vi "CSM - Read Cluster Elements From Session.vi"(5 "Section Name(\"\" as Default)":string, 8 "error in (no error)":errorcluster, 9 "Cluster":variant) -> (2 "error out":errorcluster, 3 "Cluster out":variant)   [LabVIEW 2017, in "INI-Static-Variable-Support.lvlib"]
uses:
  _Support/_fgv-oper.ctl
  99de0c97-112a-4c86-9094-c187659127e1.vi
  <userlib>/_NEVSTOP/Communicable State Machine(CSM)/addons/API-String-Arugments-Support/_Support/Data To API String Arguments.vi
  INI-Static-Variable-Support.lvlib
  <userlib>/_NEVSTOP/Communicable State Machine(CSM)/addons/API-String-Arugments-Support/API String Arguments Support.lvlib
  <vilib>/Utility/Data Type/NI_Data Type.lvlib
  <userlib>/_NEVSTOP/Communicable State Machine(CSM)/Communicable State Machine.lvlib
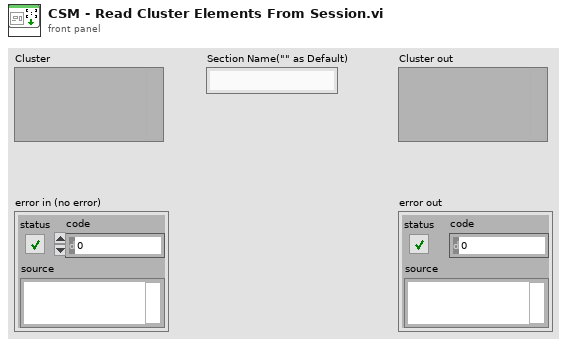
[diagram p1: front panel]
types:
  T1 = typedef "INI-Static-Variable-Support.lvlib/_fgv-oper.ctl" = enum16{"Read", "Write", "Sync", "Sessions", "List Keys", "Load", "List Files", "List Variables", "List Permanent Variables"}
  T2 = typedef "NI_Data Type.lvlib/Data Type.ctl" = enum8{"Invalid Type", "Void", "I8", "I16", "I32", "I64", "U8", "U16", "U32", "U64", "Single Float", "Double Float", "Extended Float", "Single Complex", "Double Complex", "Extended Complex", "Enum U8", "Enum U16", "Enum U32", "Enum U64", "Single Float With Unit", "Double Float With Unit", "Extended Float With Unit", "Single Complex with Unit", "Double Complex with Unit", "Extended Complex with Unit", "Boolean", "String", "Path", "Picture", "Tag", "Array", "Cluster", "Variant", "LV Variant", "Waveform", "Timestamp", "Digital Waveform", "Digital Data", "ExpressData", "Refnum", "External Data", "VI", "Poly VI", "LabVIEW Class Instance", "Fixed Point"}
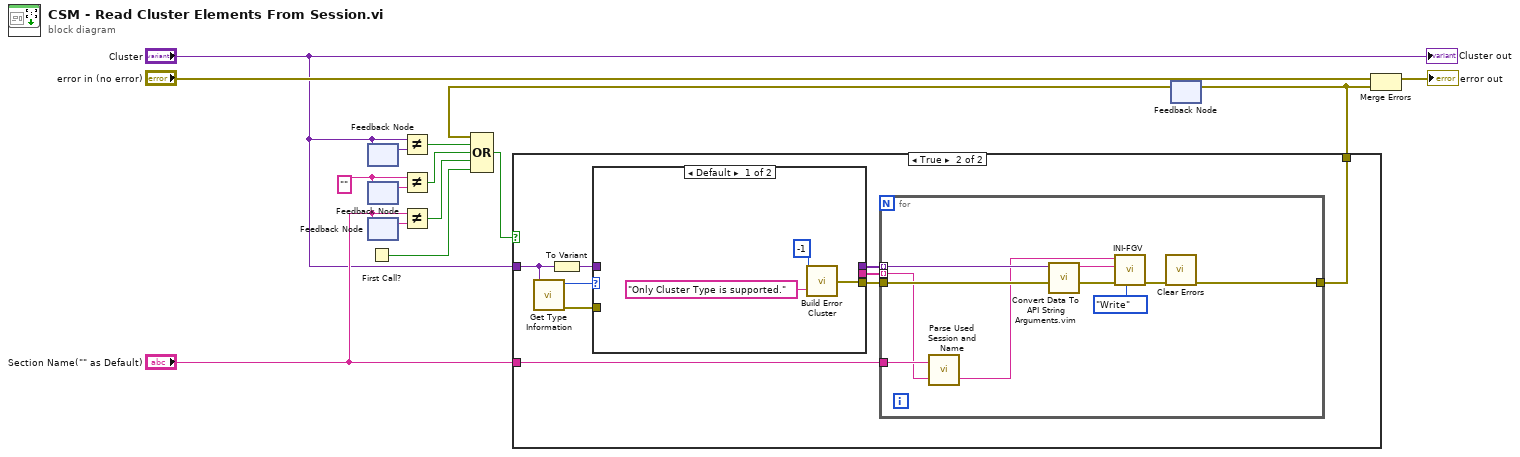
[diagram p0: block diagram]
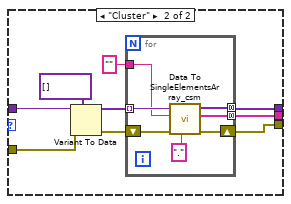
[diagram p3: hidden frame]
diagram:
  w9 = "" (">> Variable Name >>")
  n1 = First Call?() -> (First Call?: T/F=w1:bool)
  n2 = feedback #1() -> (w13:variant)  [unwired: 1 in]
  n3 = feedback-in #1("Cluster") -> ()
  n4 = feedback #2() -> (w11:string)  [unwired: 1 in]
  n5 = feedback-in #2(w9) -> ()
  n6 = feedback #3() -> (w10:string)  [unwired: 1 in]
  n7 = feedback-in #3("Section Name(\"\" as Default)") -> ()
  n8 = Not Equal?(x="Cluster", y=w13) -> (x != y?=w12:bool)
  n9 = Not Equal?(x=w9, y=w11) -> (x != y?=w7:bool)
  n10 = Not Equal?(x="Section Name(\"\" as Default)", y=w10) -> (x != y?=w6:bool)
  n11 = feedback #4() -> (w4:errorcluster)  [unwired: 1 in]
  n12 = Compound Arithmetic op=OR(w4, w12, w7, w6, w1) -> (w3:bool)
  n13 = case shown="True" w3 {
    tunnel: [_ w24] -> w5
    tunnel: "Section Name(\"\" as Default)" -> [_ w20]
    tunnel: "Cluster" -> [_ w19]
    frame False {
    }
    frame True {
      n14 = call <vilib>:"Get Type Information.vi"("Variant"=w19) -> ("error out"=w17:errorcluster, "Type"=w18:T2)  [unwired: 6 in, 3 out]
      n15 = To Variant(anything=w19) -> (Variant=w16:variant)
      n16 = case shown="Default" w18 {
        tunnel: [w26 w33] -> w23
        tunnel: [_ w32] -> w22
        tunnel: [_ w31] -> w21
        tunnel: w16 -> [_ w29]
        tunnel: w17 -> [_ w28]
        frame Default {
          n17 = call <userlib>:"Build Error Cluster.vi"("String to Prepend to source (\"\")"="Only Cluster Type is supported." ("String to Prepend to source (\"\")"), "code"=-1) -> ("error out"=w26:errorcluster)
        }
        frame "Cluster" {
          n18 = Variant To Data(error in=w28, type=variant[] [] ("Array"), Variant=w29) -> (data=w35:variant[], error out=w36:errorcluster)
          n19 = for {
            tunnel: [w42] -> w32 mode=concatenating
            tunnel: [w41] -> w31 mode=concatenating
            tunnel: w35 -> [w39] mode=indexing
            shift-right: [w40] -> w33
            shift-left: w36 -> [w38]
            tunnel: "" ("Data Name") -> [w37]
            n20 = call <userlib>:"Data To SingleElementsArray_csm.vi"("Seperator(/)"=".", "error in (no error)"=w38, "parentUrl"=w37, "Cluster"=w39) -> ("error out"=w40:errorcluster, "Full NameList"=w41:string[], "DataElementArray"=w42:variant[])  [unwired: 5 in]
          }
        }
      }
      n21 = for {
        tunnel: [w52] -> w24
        tunnel: w20 -> [w49]
        tunnel: w22 -> [w50] mode=indexing
        tunnel: w21 -> [w48] mode=indexing
        tunnel: w23 -> [w51]
        n22 = call "Parse Used Session and Name.vi"("name"=w48, "Section Name(\"\" as Default)"=w49) -> ("used name"=w47:string)  [unwired: 1 in]
        n23 = call "Convert Data To API String Arguments.vim"("error in (no error)"=w51, "data"=w50) -> ("error out"=w44:errorcluster, "String"=w45:string)  [unwired: 6 in]
        n24 = call "INI-FGV.vi"("Enum"=_fgv-oper."Write", "error IN"=w44, ">> Default Value >>"=w45, ">> Variable Name >>"=w47) -> ("error out"=w53:errorcluster)  [unwired: 5 in, 2 out]
        n25 = call <vilib>:"Clear Errors.vi"("error in (no error)"=w53) -> ("error out"=w52:errorcluster)  [unwired: 5 in, 1 out]
      }
    }
  }
  n26 = feedback-in #4(w5) -> ()
  n27 = Merge Errors("error in (no error)", w5) -> (→"error out":errorcluster)
  "Cluster out" <- "Cluster"
